vi "Array list, extract max.vi"() -> ()   [LabVIEW 2018]
panel:
  in  "배열 2":dbl[](array[numeric])
  out "배열 3":dbl[](array[numeric])
  in  "배열":dbl[](array[numeric])
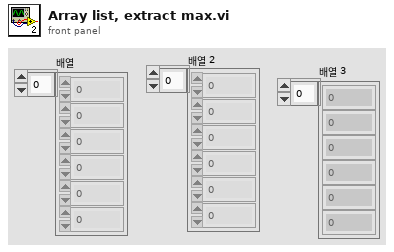
[diagram p1: front panel]
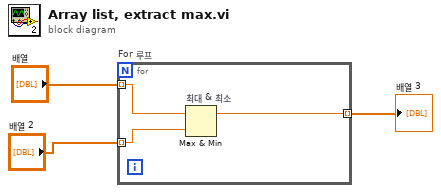
[diagram p0: block diagram]
diagram:
  n1 = for "For 루프" {
    tunnel: "배열" -> [w6] mode=indexing
    tunnel: "배열 2" -> [w5] mode=indexing
    tunnel: [w4] -> w1 mode=indexing
    n2 = Max & Min "최대 & 최소"(x=w6, y=w5) -> (max(x,y)=w4:dbl)  [unwired: 1 out]
  }
  "배열 3" <- w1
